vi "To String.Integer.Decimal.I8.vi"(1 "value":i8) -> (0 "value as string":string)   [LabVIEW 2017, in "Static Error Handling.lvlib"]
doc: "Converts the provided <B>value</B> into a decimal-formatted string."
uses:
  Static Error Handling.lvlib
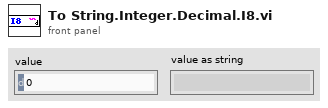
[diagram p1: front panel]
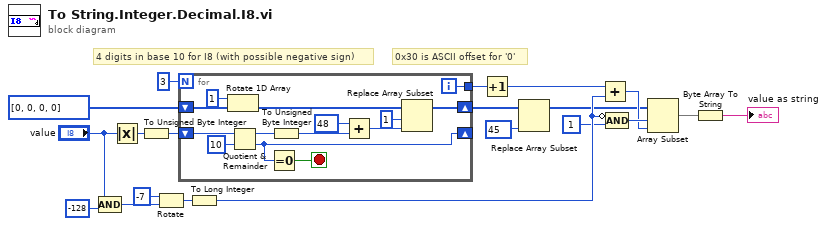
[diagram p0: block diagram]
diagram:
  # "0x30 is ASCII offset for '0'"
  # "4 digits in base 10 for I8 (with possible negative sign)"
  n1 = Compound Arithmetic op=AND("value", i8 -128 ("y")) -> (w14:i8)
  n2 = Absolute Value(x="value") -> (abs(x)=w5:i8)
  n3 = To Unsigned Byte Integer(number=w5) -> (unsigned 8bit integer=w6:u8)
  n4 = Rotate(1:w14, 2:i16 -7 ("y")) -> (0:w13:i8)
  n5 = for {
    N: 3 -> [_]
    shift-right: [w33] -> w3
    shift-left: u8[] [0, 0, 0, 0] -> [w26]
    shift-right: [w28] -> _
    shift-left: w6 -> [w30]
    tunnel: [w23] -> w16
    i -> [w23]
    stop <- w27 stop-if-true
    n6 = Rotate 1D Array(1:w26, 2:1 ("n")) -> (0:w25:u8[])
    n7 = Quotient & Remainder(x=w30, y=u8 10) -> (x-y*floor(x/y)=w29:u8, floor(x/y)=w28:u8)
    n8 = Equal To 0?(x=w28) -> (x = 0?=w27:bool)
    n9 = To Unsigned Byte Integer(number=w29) -> (unsigned 8bit integer=w22:u8)
    n10 = Add(x=u8 48 ("y"), y=w22) -> (x+y=w34:u8)
    n11 = Replace Array Subset(array=w25, new element=w34, index=1) -> (w33:u8[])
  }
  n12 = To Long Integer(number=w13) -> (32bit integer=w8:i32)
  n13 = Increment(x=w16) -> (x+1=w10:i32)
  n14 = Replace Array Subset(array=w3, new element=u8 45 ("y")) -> (w2:u8[])  [unwired: 1 in]
  n15 = Add(x=w10, y=w8) -> (x+y=w9:i32)
  n16 = Compound Arithmetic op=AND(invert w8, 1 ("y")) -> (w11:i32)
  n17 = Array Subset(array=w2, index=w11, length=w9) -> (w17:u8[])
  n18 = Byte Array To String(unsigned byte array=w17) -> (string=→"value as string":string)
